vi "一体站流程自动启动.vi"(11 "参数":T1) -> ()   [LabVIEW 2016, in "PLC.lvlib"]
uses:
  PLC.lvlib
panel:
  out "s? t:f":enum16{"初始化", "采配水启动", "仪器操作", "反冲洗", "结束"}(ring)
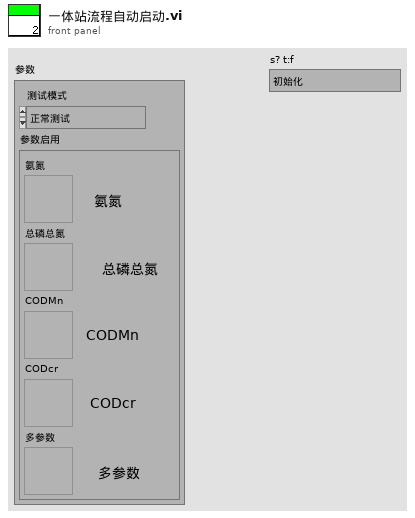
[diagram p1: front panel]
types:
  T1 = cluster{"测试模式":enum16{"正常测试", "集成干预"}, "参数启用":cluster{"氨氮":bool, "总磷总氮":bool, "CODMn":bool, "CODcr":bool, "多参数":bool}}
  T2 = cluster{"命令":string, cluster{"starting address":u16, "holding register value":u16}}
  T3 = enum16{"启动测量", "标样核查", "零点核查", "跨度核查", "空白测试", "平行样测试", "加标回收", "空白校准", "标样校准", "初始化（清洗）", "停止测试", "仪器重启", "校时", "模式设置", "测量间隔设置"}
  T4 = cluster{"时间标识":timestamp, "设备":string, "日志信息":string, "流程参数":string}
  T5 = cluster{"测量模式":enum16{"水样测量", "标样核查", "零点核查", "跨度核查", "空白测试", "加标回收", "平行样", "校零", "校标"}}
  T6 = cluster{"时间标识":timestamp, "设备":string, "日志信息":string}
  T7 = enum16{"空闲", "水样测试", "标样核查", "零点核查", "跨度核查", "空白测试", "平行样测试", "加标回收", "空白校准", "标样校准", "初始化（清洗）"}
  T8 = cluster{"R0":i16, "R1":i16, "R2":i16, "R3":i16, "R4":i16, "R5":i16, "R6":i16, "R7":i16, "R8":i16, "R9":i16, "R10":i16, "R11":i16, "R12":i16, "R13":i16, "R14":i16, "R15":i16, "R16":i16, "R17":i16, "R18":i16, "R19":i16, "R20":i16, "R21":i16, "R22":i16, "R23":i16, "R24":i16, "R25":i16, "R26":i16, "R27":i16, "R28":i16, "R29":i16, "R30":i16, "R31":i16, "R32":i16, "R33":i16, "R34":i16, "R35":i16, "R36":i16, "R37":i16, "R38":i16, "R39":i16, "R40":i16, "R41":i16, "R42":i16, "R43":i16, "R44":i16, "R45":i16, "R46":i16, "R47":i16, "R48":i16, "R49":i16, "R50":i16, "R51":i16, "R52":i16, "R53":i16, "R54":i16, "R55":i16, "R56":i16}
  T9 = cluster{"R100":i16, "R101":i16, "R102":i16, "R103":i16, "R104":i16, "R105":i16, "R106":i16, "R107":i16, "R108":i16, "R109":i16, "R110":i16, "R111":i16, "R112":i16, "R113":i16, "R114":i16, "R115":i16, "R116":i16, "R117":i16, "R118":i16, "R119":i16, "R120":i16, "R121":i16, "R122":i16, "R123":i16}
  T10 = enum32{"Bad", "Idle", "Run top level", "Running"}
  T11 = cluster{"氨氮":bool, "总磷总氮":bool, "CODMn":bool, "CODcr":bool, "多参数":bool}
  T12 = cluster{"时间标识":timestamp, "参数":string, "数据类型":string, "集成干预测试浓度值":dbl, "集成干预前测试时间":timestamp, "集成干预前测试浓度值":dbl}
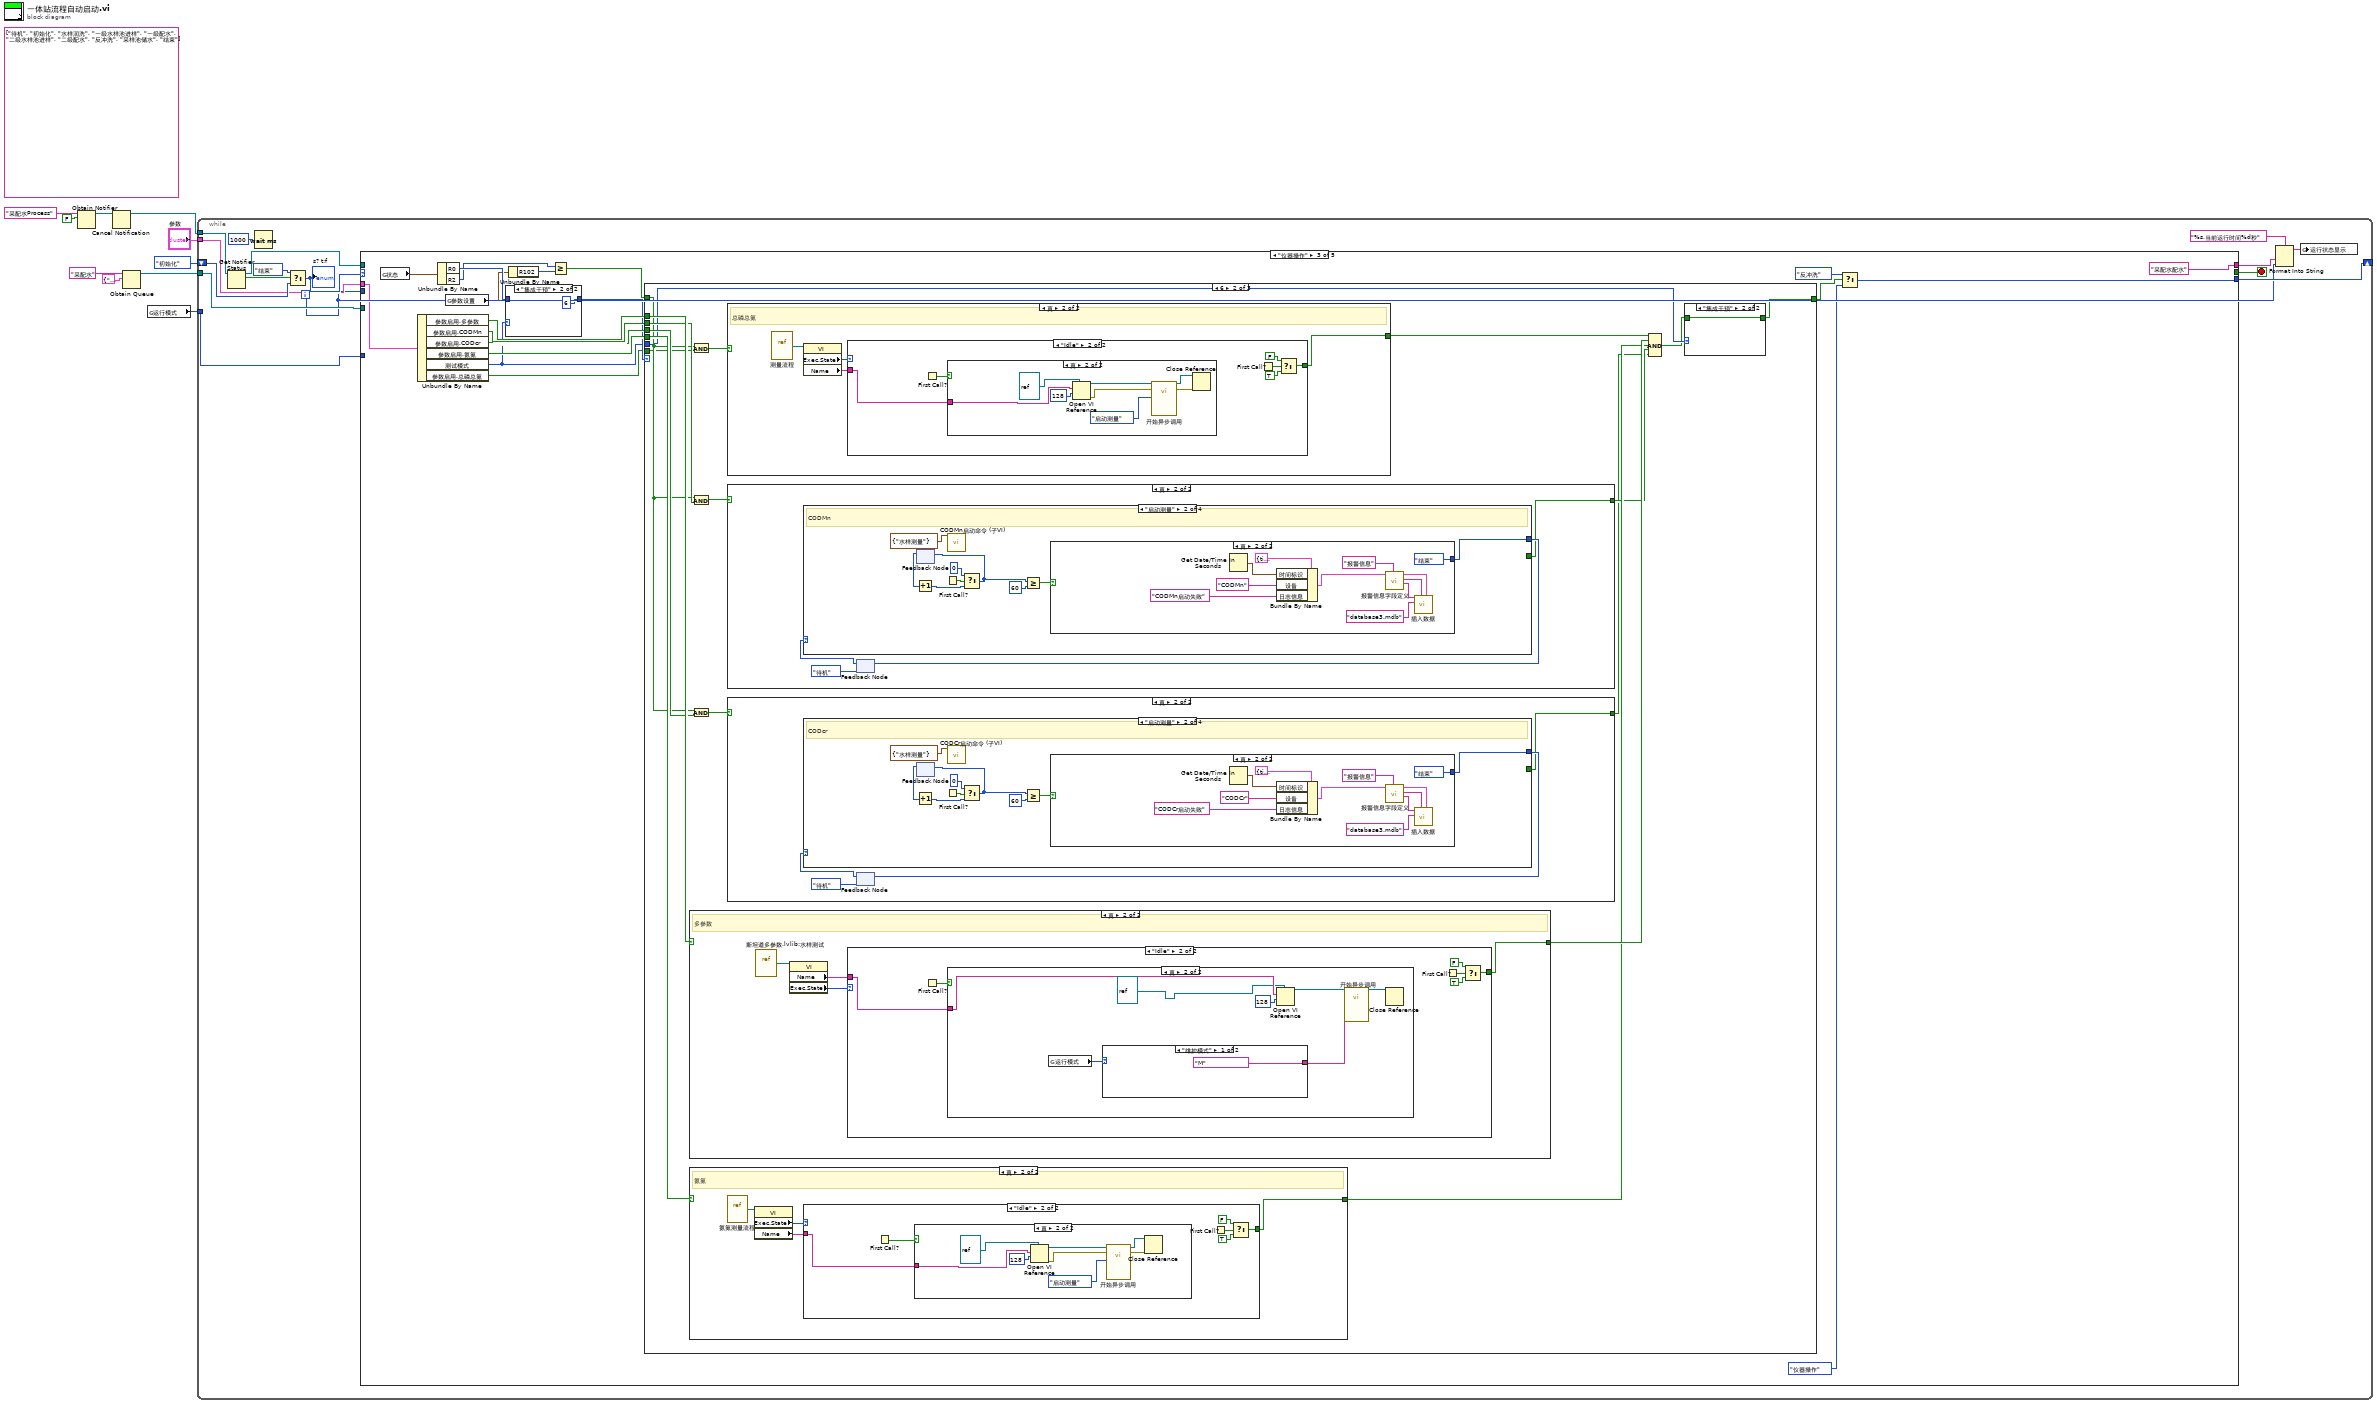
[diagram p0: block diagram]
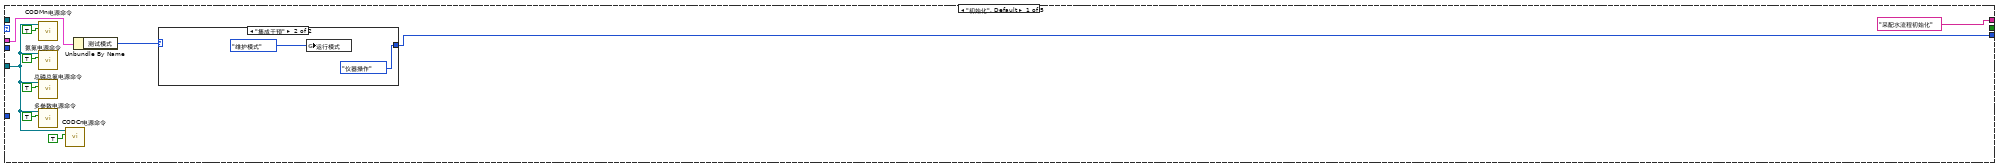
[diagram p2: hidden frame]
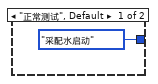
[diagram p3: hidden frame]
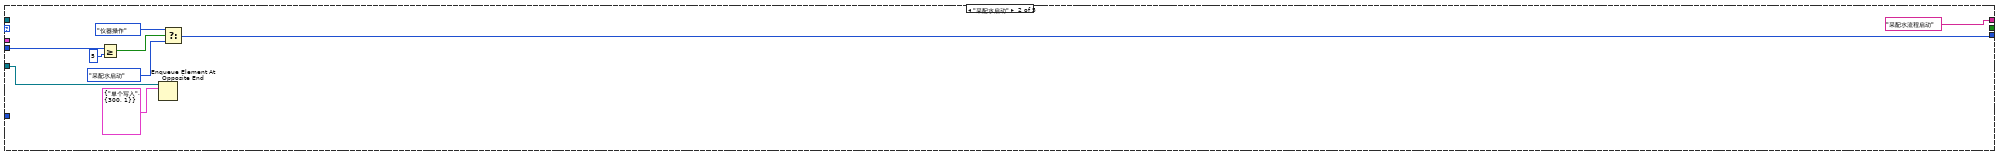
[diagram p4: hidden frame]
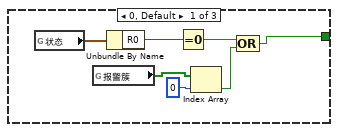
[diagram p6: hidden frame]
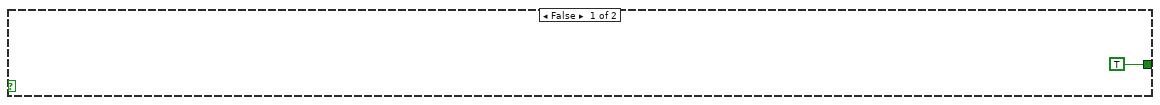
[diagram p7: hidden frame]
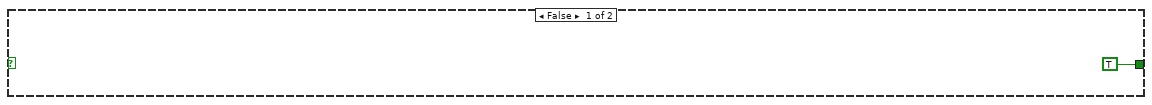
[diagram p11: hidden frame]
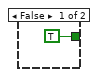
[diagram p14: hidden frame]
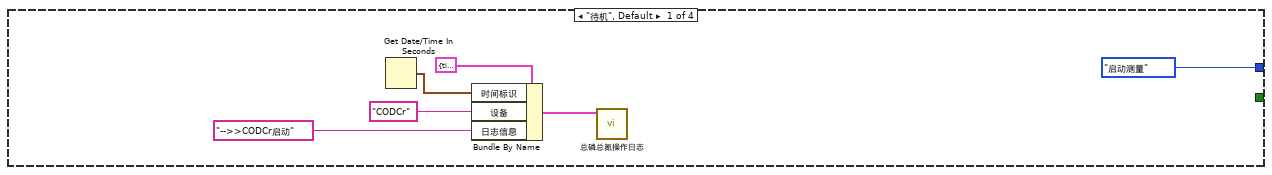
[diagram p15: hidden frame]
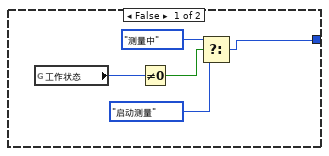
[diagram p16: hidden frame]
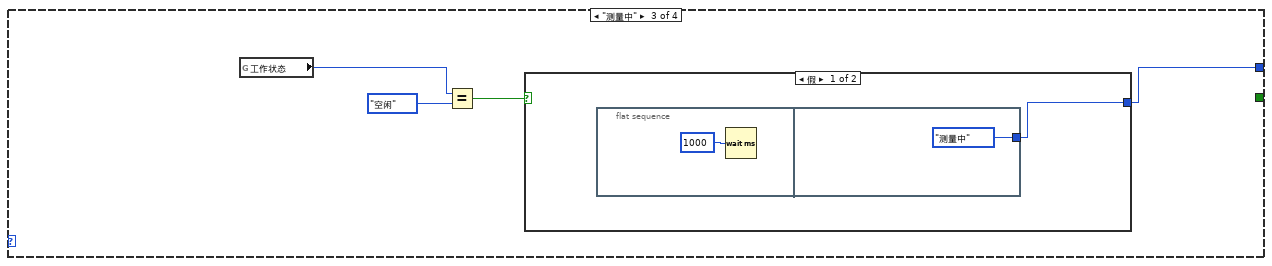
[diagram p17: hidden frame]
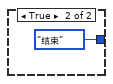
[diagram p18: hidden frame]
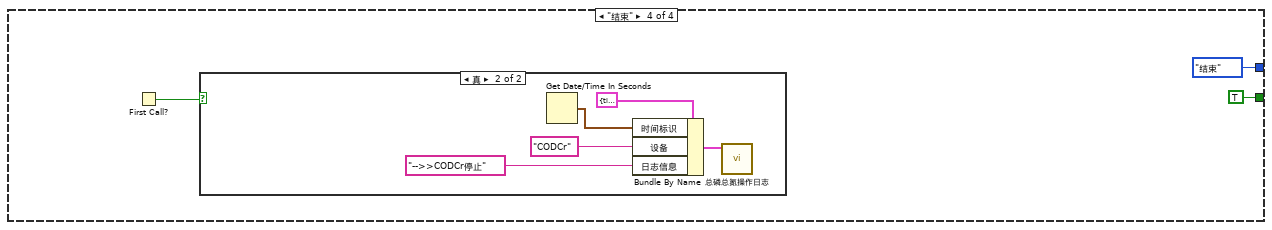
[diagram p19: hidden frame]
diagram:
  (unwired) string[][] [["待机"], ["初始化"], ["水样润洗"], ["一级水样池进样"], ["一级配水"], ["二级水样池进样"], ["二级配水"], ["反冲洗"], ["采样池储水"], ["结束"]] ("项名")
  n1 = Obtain Notifier(name (unnamed)="采配水Process" ("名称（未命名）"), notification data type=FALSE) -> (notifier out=w4:refnum<notifier>)  [unwired: 2 in, 2 out]
  n2 = Cancel Notification(0:w4) -> (8:w3:refnum<notifier>)  [unwired: 1 in, 2 out]
  n3 = Obtain Queue(name (unnamed)="采配水" ("名称（未命名）"), element data type=cluster{"命令":string, "数据":variant} {"命令"="", "数据"=variant}) -> (queue out=w7:refnum<queue>)  [unwired: 3 in, 2 out]
  n4 = global read "系统设置全局变量.vi" "运行模式"() -> (w1:enum16{"维护模式", "常规模式", "应急模式", "质控模式"})
  n5 = while {
    shift-right: [w23] -> _
    shift-left: enum16{"初始化", "采配水启动", "仪器操作", "反冲洗", "结束"}."初始化" ("枚举") -> [w19]
    tunnel: w7 -> [w26]
    tunnel: w3 -> [w22]
    tunnel: "参数" -> [w13]
    tunnel: w1 -> [w12]
    i -> [w11]
    stop <- w25 stop-if-true
    n6 = Get Notifier Status(notifier=w22) -> (notifier out=w14:refnum<notifier>, current notification=w21:bool)  [unwired: 1 in, 3 out]
    n7 = Wait (ms)(milliseconds to wait=u32 1000 ("等待时间（毫秒）")) -> ()  [unwired: 1 out]
    n8 = Select(t=enum16{"初始化", "采配水启动", "仪器操作", "反冲洗", "结束"}."结束" ("枚举"), s=w21, f=w19) -> (s? t:f=w18:enum16{"初始化", "采配水启动", "仪器操作", "反冲洗", "结束"})
    "s? t:f" <- w18
    n9 = case shown="\"仪器操作\"" w18 {
      tunnel: w26 -> [w31 w48 _ _ w434]
      tunnel: [_ _ _ _ TRUE] -> w25
      tunnel: [w30 w40 w62 w261 enum16{"初始化", "采配水启动", "仪器操作", "反冲洗", "结束"}."结束" ("枚举")] -> w23
      tunnel: ["采配水流程初始化" "采配水流程启动" "采配水配水" "等待测试完成" "采配水结束"] -> w15
      tunnel: w14 -> [_ _ _ _ w435]
      tunnel: w13 -> [w28 _ w65 w260 w431]
      tunnel: w12 -> [_ _ _ w257 w430]
      tunnel: w11 -> [_ w46 _ _ _]
      frame "初始化", Default {
        n10 = call "CODMn电源命令.vi"("通电/断电"=TRUE, "队列"=w31) -> ()  [unwired: 9 in, 1 out]
        n11 = call "氨氮电源命令.vi"("通电/断电"=TRUE, "队列"=w31) -> ()  [unwired: 9 in, 1 out]
        n12 = call "总磷总氮电源命令.vi"("通电/断电"=TRUE, "队列"=w31) -> ()  [unwired: 9 in, 1 out]
        n13 = call "多参数电源命令.vi"("通电/断电"=TRUE, "队列"=w31) -> ()  [unwired: 9 in, 1 out]
        n14 = call "CODCr电源命令.vi"("通电/断电"=TRUE, "队列"=w31) -> ()  [unwired: 9 in, 1 out]
        n15 = Unbundle By Name(w28) -> ("测试模式"=w27:enum16{"正常测试", "集成干预"})
        n16 = case shown="\"集成干预\"" w27 {
          tunnel: [enum16{"初始化", "采配水启动", "仪器操作", "反冲洗", "结束"}."采配水启动" ("枚举") enum16{"初始化", "采配水启动", "仪器操作", "反冲洗", "结束"}."仪器操作" ("枚举")] -> w30
          frame "正常测试", Default {
          }
          frame "集成干预" {
            n17 = global write "系统设置全局变量.vi" "运行模式"(enum16{"维护模式", "常规模式", "应急模式", "质控模式"}."维护模式" ("运行模式")) -> ()
          }
        }
      }
      frame "采配水启动" {
        n18 = Greater Or Equal?(x=w46, y=5) -> (x >= y?=w43:bool)
        n19 = Enqueue Element At Opposite End(queue=w48, element=T2 {"命令"="单个写入", {"starting address"=300, "holding register value"=1}} ("元素")) -> ()  [unwired: 2 in, 3 out]
        n20 = Select(t=enum16{"初始化", "采配水启动", "仪器操作", "反冲洗", "结束"}."仪器操作" ("枚举"), s=w43, f=enum16{"初始化", "采配水启动", "仪器操作", "反冲洗", "结束"}."采配水启动" ("枚举")) -> (s? t:f=w40:enum16{"初始化", "采配水启动", "仪器操作", "反冲洗", "结束"})
      }
      frame "仪器操作" {
        n21 = global read "采配水全局变量.vi" "状态"() -> (w67:T8)
        n22 = Unbundle By Name(w65) -> ("参数启用.多参数"=w60:bool, "参数启用.CODMn"=w59:bool, "参数启用.CODcr"=w58:bool, "参数启用.氨氮"=w57:bool, "测试模式"=w50:enum16{"正常测试", "集成干预"}, "参数启用.总磷总氮"=w49:bool)
        n23 = Unbundle By Name(w67) -> ("R0"=w56:i16, "R2"=w51:i16)
        n24 = global read "采配水全局变量.vi" "参数设置"() -> (w53:T9)
        n25 = case shown="\"集成干预\"" w50 {
          tunnel: w56 -> [w68 _]
          tunnel: [w68 i16 6 ("R0")] -> w55
          frame "正常测试", Default {
          }
          frame "集成干预" {
          }
        }
        n26 = Unbundle By Name(w53) -> ("R102"=w54:i16)
        n27 = Greater Or Equal?(x=w51, y=w54) -> (x >= y?=w52:bool)
        n28 = case shown="6" w55 {
          tunnel: [w71 w81 TRUE] -> w64
          tunnel: w60 -> [_ w93 _]
          tunnel: w59 -> [_ w92 _]
          tunnel: w58 -> [_ w89 _]
          tunnel: w57 -> [_ w88 _]
          tunnel: w52 -> [_ w80 _]
          tunnel: w50 -> [_ w83 _]
          tunnel: w49 -> [_ w79 _]
          frame 0, Default {
            n29 = global read "采配水全局变量.vi" "状态"() -> (w74:T8)
            n30 = global read "采配水全局变量.vi" "报警簇"() -> (w75:bool[])
            n31 = Unbundle By Name(w74) -> ("R0"=w73:i16)
            n32 = Equal To 0?(x=w73) -> (x = 0?=w76:bool)
            n33 = Index Array(array=w75, index=0 ("索引")) -> (element=w70:bool)
            n34 = Compound Arithmetic op=OR ("复合运算")(w76, w70) -> (w71:bool)
          }
          frame 6 {
            n35 = case shown="真" w93 {
              tunnel: [TRUE ("t") w237] -> w87
              frame False {
              }
              frame True {
                # "多参数"
                n36 = vi-ref "斯坦道多参数.lvlib:水样测试.vi"() -> (w239:refnum<vi>)
                n37 = property class="VI"(reference=w239) -> ("Name"=w238:string, "Exec.State"=w240:T10)  [unwired: 1 in, 2 out]
                n38 = case shown="\"Idle\"" w240 {
                  tunnel: w238 -> [_ w246]
                  tunnel: [_ w241] -> w237
                  frame "Bad", Default {
                  }
                  frame "Idle" {
                    n39 = First Call?() -> (First Call?: T/F=w245:bool)
                    n40 = case shown="真" w245 {
                      tunnel: w246 -> [_ w252]
                      frame False {
                      }
                      frame True {
                        n41 = global read "系统设置全局变量.vi" "运行模式"() -> (w249:enum16{"维护模式", "常规模式", "应急模式", "质控模式"})
                        n42 = case shown="\"维护模式\"" w249 {
                          tunnel: ["M" ("数据标记表") "N" ("数据标记表")] -> w248
                          frame "维护模式" {
                          }
                          frame "常规模式", Default {
                          }
                        }
                        n43 = Open VI Reference(type specifier VI Refnum (for type only)=refnum<vi> refnum, vi path=w252, options=128 ("选项")) -> (vi reference=w251:refnum<vi>)  [unwired: 3 in, 1 out]
                        n44 = call-by-ref "开始异步调用"(reference=w251, "数据标记表"=w248) -> (reference out=w250:refnum<vi>)  [unwired: 12 in, 1 out]
                        n45 = Close Reference(reference=w250) -> ()  [unwired: 1 in, 1 out]
                      }
                    }
                    n46 = First Call?() -> (First Call?: T/F=w244:bool)
                    n47 = Select(t=FALSE, s=w244, f=TRUE) -> (s? t:f=w241:bool)
                  }
                }
              }
            }
            n48 = case "条件结构" shown="真" w88 {
              tunnel: [TRUE ("t") w115] -> w86
              frame False {
              }
              frame True {
                # "氨氮"
                n49 = vi-ref "氨氮测量流程.vi"() -> (w118:refnum<vi>)
                n50 = property class="VI"(reference=w118) -> ("Exec.State"=w117:T10, "Name"=w116:string)  [unwired: 1 in, 2 out]
                n51 = case shown="\"Idle\"" w117 {
                  tunnel: w116 -> [_ w124]
                  tunnel: [_ w119] -> w115
                  frame "Bad", Default {
                  }
                  frame "Idle" {
                    n52 = First Call?() -> (First Call?: T/F=w123:bool)
                    n53 = case shown="真" w123 {
                      tunnel: w124 -> [_ w129]
                      frame False {
                      }
                      frame True {
                        n54 = Open VI Reference(type specifier VI Refnum (for type only)=refnum<vi> refnum, vi path=w129, options=128 ("选项")) -> (vi reference=w127:refnum<vi>, error out=w130:errorcluster)  [unwired: 3 in]
                        n55 = call-by-ref "开始异步调用"(reference=w127, error in=w130, "控制命令"=T3."启动测量") -> (reference out=w131:refnum<vi>, error out=w132:errorcluster)  [unwired: 11 in]
                        n56 = Close Reference(reference=w131, error in (no error)=w132) -> ()  [unwired: 1 out]
                      }
                    }
                    n57 = First Call?() -> (First Call?: T/F=w122:bool)
                    n58 = Select(t=FALSE, s=w122, f=TRUE) -> (s? t:f=w119:bool)
                  }
                }
              }
            }
            n59 = And(x=w80, y=w79) -> (x .and. y?=w78:bool)
            n60 = And(x=w80, y=w92) -> (x .and. y?=w91:bool)
            n61 = And(x=w80, y=w89) -> (x .and. y?=w90:bool)
            n62 = case "条件结构" shown="真" w78 {
              tunnel: [TRUE ("t") w95] -> w77
              frame False {
              }
              frame True {
                # "总磷总氮"
                n63 = vi-ref "测量流程.vi"() -> (w98:refnum<vi>)
                n64 = property class="VI"(reference=w98) -> ("Exec.State"=w97:T10, "Name"=w96:string)  [unwired: 1 in, 2 out]
                n65 = case shown="\"Idle\"" w97 {
                  tunnel: w96 -> [_ w104]
                  tunnel: [_ w99] -> w95
                  frame "Bad", Default {
                  }
                  frame "Idle" {
                    n66 = First Call?() -> (First Call?: T/F=w103:bool)
                    n67 = case shown="真" w103 {
                      tunnel: w104 -> [_ w109]
                      frame False {
                      }
                      frame True {
                        n68 = Open VI Reference(type specifier VI Refnum (for type only)=refnum<vi> refnum, vi path=w109, options=128 ("选项")) -> (vi reference=w107:refnum<vi>, error out=w110:errorcluster)  [unwired: 3 in]
                        n69 = call-by-ref "开始异步调用"(reference=w107, error in=w110, "控制命令"=T3."启动测量") -> (reference out=w111:refnum<vi>, error out=w112:errorcluster)  [unwired: 11 in]
                        n70 = Close Reference(reference=w111, error in (no error)=w112) -> ()  [unwired: 1 out]
                      }
                    }
                    n71 = First Call?() -> (First Call?: T/F=w102:bool)
                    n72 = Select(t=FALSE, s=w102, f=TRUE) -> (s? t:f=w99:bool)
                  }
                }
              }
            }
            n73 = case shown="真" w91 {
              tunnel: [TRUE w186] -> w85
              frame False {
              }
              frame True {
                n74 = feedback #1(enum16{"待机", "启动测量", "测量中", "结束"}."待机") -> (w188:enum16{"待机", "启动测量", "测量中", "结束"})
                n75 = case shown="\"启动测量\"" w188 {
                  tunnel: [enum16{"待机", "启动测量", "测量中", "结束"}."启动测量" w204 w223 enum16{"待机", "启动测量", "测量中", "结束"}."结束"] -> w187
                  tunnel: [_ _ _ TRUE] -> w186
                  frame "待机", Default {
                    n76 = Get Date/Time In Seconds() -> (seconds since 1Jan1904=w194:timestamp)
                    n77 = Bundle By Name(cluster=T4 {"时间标识"=timestamp(0 s since 1904-01-01), "设备"="", "日志信息"="", "流程参数"=""} ("data in"), "时间标识"=w194, "设备"="CODMn", "日志信息"="-->>CODMn启动") -> (w190:T4)
                    n78 = call "总磷总氮操作日志.vi"("data in"=w190) -> ()  [unwired: 11 in]
                  }
                  frame "启动测量" {
                    # "CODMn"
                    n79 = feedback #2() -> (w200:i32)  [unwired: 1 in]
                    n80 = Increment(x=w200) -> (x+1=w201:i32)
                    n81 = First Call?() -> (First Call?: T/F=w199:bool)
                    n82 = call "CODMn启动命令 (子VI).vi"("启动测量模式"=T5 {"测量模式"=enum."水样测量"}) -> ()  [unwired: 11 in]
                    n83 = Select(t=0, s=w199, f=w201) -> (s? t:f=w202:i32)
                    n84 = feedback-in #2(w202) -> ()
                    n85 = Greater Or Equal?(x=w202, y=60) -> (x >= y?=w197:bool)
                    n86 = case shown="真" w197 {
                      tunnel: [w206 enum16{"待机", "启动测量", "测量中", "结束"}."结束"] -> w204
                      frame False {
                        n87 = global read "运行时序全局变量.vi" "多列列表框"() -> (w205:i32)
                        n88 = Not Equal To 0?(x=w205) -> (x != 0?=w207:bool)
                        n89 = Select(t=enum16{"待机", "启动测量", "测量中", "结束"}."测量中", s=w207, f=enum16{"待机", "启动测量", "测量中", "结束"}."启动测量") -> (s? t:f=w206:enum16{"待机", "启动测量", "测量中", "结束"})
                      }
                      frame True {
                        n90 = Get Date/Time In Seconds() -> (seconds since 1Jan1904=w216:timestamp)
                        n91 = Bundle By Name(cluster=T6 {"时间标识"=timestamp(0 s since 1904-01-01), "设备"="", "日志信息"=""} ("data in"), "时间标识"=w216, "设备"="CODMn", "日志信息"="CODMn启动失败") -> (w210:T6)
                        n92 = call "报警信息字段定义.vi"("table输入"="报警信息", "data in"=w210) -> ("table输出"=w213:string, "columns"=w214:string[], "data out"=w215:T6)  [unwired: 7 in]
                        n93 = call "插入数据.vi"("data"=w215, "columns"=w214, "database"="database3.mdb", "table"=w213) -> ()  [unwired: 7 in, 1 out]
                      }
                    }
                  }
                  frame "测量中" {
                    n94 = global read "运行时序全局变量.vi" "多列列表框"() -> (w222:i32)
                    n95 = Equal To 0?(x=w222) -> (x = 0?=w221:bool)
                    n96 = case shown="假" w221 {
                      tunnel: [w224 enum16{"待机", "启动测量", "测量中", "结束"}."结束"] -> w223
                      frame False {
                        n97 = flat-sequence {
                          tunnel: [enum16{"待机", "启动测量", "测量中", "结束"}."测量中"] -> w224
                          frame #0 {
                            n98 = Wait (ms)(milliseconds to wait=u32 1000 ("等待时间（毫秒）")) -> ()  [unwired: 1 out]
                          }
                          frame #1 {
                          }
                        }
                      }
                      frame True {
                      }
                    }
                  }
                  frame "结束" {
                    n99 = First Call?() -> (First Call?: T/F=w228:bool)
                    n100 = case shown="真" w228 {
                      frame False {
                      }
                      frame True {
                        n101 = Get Date/Time In Seconds() -> (seconds since 1Jan1904=w235:timestamp)
                        n102 = Bundle By Name(cluster=T4 {"时间标识"=timestamp(0 s since 1904-01-01), "设备"="", "日志信息"="", "流程参数"=""} ("data in"), "时间标识"=w235, "设备"="CODMn", "日志信息"="-->>CODMn停止") -> (w231:T4)
                        n103 = call "总磷总氮操作日志.vi"("data in"=w231) -> ()  [unwired: 11 in]
                      }
                    }
                  }
                }
                n104 = feedback-in #1(w187) -> ()
              }
            }
            n105 = case shown="真" w90 {
              tunnel: [TRUE w134] -> w84
              frame False {
              }
              frame True {
                n106 = feedback #3(enum16{"待机", "启动测量", "测量中", "结束"}."待机") -> (w136:enum16{"待机", "启动测量", "测量中", "结束"})
                n107 = case shown="\"启动测量\"" w136 {
                  tunnel: [enum16{"待机", "启动测量", "测量中", "结束"}."启动测量" w152 w172 enum16{"待机", "启动测量", "测量中", "结束"}."结束"] -> w135
                  tunnel: [_ _ _ TRUE] -> w134
                  frame "待机", Default {
                    n108 = Get Date/Time In Seconds() -> (seconds since 1Jan1904=w142:timestamp)
                    n109 = Bundle By Name(cluster=T4 {"时间标识"=timestamp(0 s since 1904-01-01), "设备"="", "日志信息"="", "流程参数"=""} ("data in"), "时间标识"=w142, "设备"="CODCr", "日志信息"="-->>CODCr启动") -> (w138:T4)
                    n110 = call "总磷总氮操作日志.vi"("data in"=w138) -> ()  [unwired: 11 in]
                  }
                  frame "启动测量" {
                    # "CODcr"
                    n111 = feedback #4() -> (w148:i32)  [unwired: 1 in]
                    n112 = Increment(x=w148) -> (x+1=w149:i32)
                    n113 = First Call?() -> (First Call?: T/F=w147:bool)
                    n114 = call "CODCr启动命令 (子VI).vi"("启动测量模式"=T5 {"测量模式"=enum."水样测量"}) -> ()  [unwired: 11 in]
                    n115 = Select(t=0, s=w147, f=w149) -> (s? t:f=w150:i32)
                    n116 = feedback-in #4(w150) -> ()
                    n117 = Greater Or Equal?(x=w150, y=60) -> (x >= y?=w145:bool)
                    n118 = case shown="真" w145 {
                      tunnel: [w153 enum16{"待机", "启动测量", "测量中", "结束"}."结束"] -> w152
                      frame False {
                        n119 = global read "CODcr全局变量.vi" "工作状态"() -> (w154:T7)
                        n120 = Not Equal To 0?(x=w154) -> (x != 0?=w155:bool)
                        n121 = Select(t=enum16{"待机", "启动测量", "测量中", "结束"}."测量中", s=w155, f=enum16{"待机", "启动测量", "测量中", "结束"}."启动测量") -> (s? t:f=w153:enum16{"待机", "启动测量", "测量中", "结束"})
                      }
                      frame True {
                        n122 = Get Date/Time In Seconds() -> (seconds since 1Jan1904=w164:timestamp)
                        n123 = Bundle By Name(cluster=T6 {"时间标识"=timestamp(0 s since 1904-01-01), "设备"="", "日志信息"=""} ("data in"), "时间标识"=w164, "设备"="CODCr", "日志信息"="CODCr启动失败") -> (w158:T6)
                        n124 = call "报警信息字段定义.vi"("table输入"="报警信息", "data in"=w158) -> ("table输出"=w161:string, "columns"=w162:string[], "data out"=w163:T6)  [unwired: 7 in]
                        n125 = call "插入数据.vi"("data"=w163, "columns"=w162, "database"="database3.mdb", "table"=w161) -> ()  [unwired: 7 in, 1 out]
                      }
                    }
                  }
                  frame "测量中" {
                    n126 = global read "CODcr全局变量.vi" "工作状态"() -> (w171:T7)
                    n127 = Equal?(x=w171, y=T7."空闲" ("工作状态")) -> (x = y?=w170:bool)
                    n128 = case shown="假" w170 {
                      tunnel: [w173 enum16{"待机", "启动测量", "测量中", "结束"}."结束"] -> w172
                      frame False {
                        n129 = flat-sequence {
                          tunnel: [enum16{"待机", "启动测量", "测量中", "结束"}."测量中"] -> w173
                          frame #0 {
                            n130 = Wait (ms)(milliseconds to wait=u32 1000 ("等待时间（毫秒）")) -> ()  [unwired: 1 out]
                          }
                          frame #1 {
                          }
                        }
                      }
                      frame True {
                      }
                    }
                  }
                  frame "结束" {
                    n131 = First Call?() -> (First Call?: T/F=w177:bool)
                    n132 = case shown="真" w177 {
                      frame False {
                      }
                      frame True {
                        n133 = Get Date/Time In Seconds() -> (seconds since 1Jan1904=w184:timestamp)
                        n134 = Bundle By Name(cluster=T4 {"时间标识"=timestamp(0 s since 1904-01-01), "设备"="", "日志信息"="", "流程参数"=""} ("data in"), "时间标识"=w184, "设备"="CODCr", "日志信息"="-->>CODCr停止") -> (w180:T4)
                        n135 = call "总磷总氮操作日志.vi"("data in"=w180) -> ()  [unwired: 11 in]
                      }
                    }
                  }
                }
                n136 = feedback-in #3(w135) -> ()
              }
            }
            n137 = Compound Arithmetic op=AND ("复合运算")(w77, w87, w86, w85, w84) -> (w82:bool)
            n138 = case shown="\"集成干预\"" w83 {
              tunnel: w82 -> [_ w113]
              tunnel: [_ w113] -> w81
              frame "正常测试", Default {
              }
              frame "集成干预" {
              }
            }
          }
          frame 7..9 {
          }
        }
        n139 = Select(t=enum16{"初始化", "采配水启动", "仪器操作", "反冲洗", "结束"}."反冲洗" ("枚举"), s=w64, f=enum16{"初始化", "采配水启动", "仪器操作", "反冲洗", "结束"}."仪器操作" ("枚举")) -> (s? t:f=w62:enum16{"初始化", "采配水启动", "仪器操作", "反冲洗", "结束"})
      }
      frame "反冲洗" {
        n140 = First Call?() -> (First Call?: T/F=w258:bool)
        n141 = case shown="真" w258 {
          tunnel: w260 -> [_ w270]
          tunnel: w257 -> [_ w267]
          frame False {
          }
          frame True {
            n142 = Unbundle By Name(w270) -> ("测试模式"=w269:enum16{"正常测试", "集成干预"}, "参数启用"=w268:T11)
            n143 = case shown="\"集成干预\"" w269 {
              tunnel: w268 -> [w273 w358]
              tunnel: w267 -> [_ w353]
              frame "正常测试", Default {
                n144 = global read "系统设置全局变量.vi" "运行模式"() -> (w271:enum16{"维护模式", "常规模式", "应急模式", "质控模式"})
                n145 = global read "采配水全局变量.vi" "报警簇"() -> (w278:bool[])
                n146 = case shown="\"维护模式\"" w271 {
                  tunnel: ["M" ("table") "N" ("table")] -> w272
                  frame "维护模式" {
                  }
                  frame "常规模式", Default {
                  }
                }
                n147 = Index Array(array=w278, index #1=0 ("索引"), index #2=11 ("索引")) -> (element #1=w275:bool, element #2=w274:bool)
                n148 = case shown="假" w275 {
                  tunnel: w274 -> [w284 _]
                  tunnel: w273 -> [w283 w297]
                  tunnel: w272 -> [w281 w291]
                  frame False {
                    n149 = Unbundle By Name(w283) -> ("氨氮"=w282:bool)
                    n150 = case shown="真" w284 {
                      tunnel: w282 -> [_ w286]
                      tunnel: w281 -> [_ w285]
                      frame False {
                      }
                      frame True {
                        n151 = case shown="真" w286 {
                          tunnel: w285 -> [_ w287]
                          tunnel: [_ w288] -> _
                          frame False {
                          }
                          frame True {
                            n152 = call "取水点无水样数据存储.vi"("数据标识"="lw", "数据类型"=w287, "table"="氨氮") -> ("error out"=w288:errorcluster)  [unwired: 8 in]
                          }
                        }
                      }
                    }
                  }
                  frame True {
                    n153 = Unbundle By Name(w297) -> ("氨氮"=w296:bool, "CODMn"=w295:bool, "CODcr"=w294:bool, "多参数"=w293:bool, "总磷总氮"=w292:bool)
                    n154 = case shown="真" w296 {
                      tunnel: w291 -> [_ w349]
                      tunnel: [_ w350] -> _
                      frame False {
                      }
                      frame True {
                        n155 = call "取水点无水样数据存储.vi"("数据标识"="Z", "数据类型"=w349, "table"="氨氮") -> ("error out"=w350:errorcluster)  [unwired: 8 in]
                      }
                    }
                    n156 = case shown="真" w295 {
                      tunnel: w291 -> [_ w346]
                      tunnel: [_ w345] -> _
                      frame False {
                      }
                      frame True {
                        n157 = call "取水点无水样数据存储.vi"("数据标识"="Z", "数据类型"=w346, "table"="CODMn") -> ("error out"=w345:errorcluster)  [unwired: 8 in]
                      }
                    }
                    n158 = case shown="真" w294 {
                      tunnel: w291 -> [_ w342]
                      tunnel: [_ w341] -> _
                      frame False {
                      }
                      frame True {
                        n159 = call "取水点无水样数据存储.vi"("数据标识"="Z", "数据类型"=w342, "table"="CODCr") -> ("error out"=w341:errorcluster)  [unwired: 8 in]
                      }
                    }
                    n160 = case shown="真" w292 {
                      tunnel: w291 -> [_ w299]
                      tunnel: [_ w298] -> _
                      frame False {
                      }
                      frame True {
                        n161 = call "取水点无水样数据存储.vi"("数据标识"="Z", "数据类型"=w299, "table"="总氮") -> ("error out"=w300:errorcluster)  [unwired: 8 in]
                        n162 = call "取水点无水样数据存储.vi"("error in (no error)"=w300, "数据标识"="Z", "数据类型"=w299, "table"="总磷") -> ("error out"=w298:errorcluster)  [unwired: 7 in]
                      }
                    }
                    n163 = case shown="真" w293 {
                      tunnel: w291 -> [_ w312]
                      frame False {
                      }
                      frame True {
                        n164 = global read "断电保存变量.vi" "Cond"() -> (w307:bool)
                        n165 = global read "断电保存变量.vi" "Turb"() -> (w308:bool)
                        n166 = global read "断电保存变量.vi" "DO"() -> (w309:bool)
                        n167 = global read "断电保存变量.vi" "pH"() -> (w310:bool)
                        n168 = global read "断电保存变量.vi" "藻密度"() -> (w306:bool)
                        n169 = global read "断电保存变量.vi" "Temp"() -> (w311:bool)
                        n170 = case shown="真" w310 {
                          tunnel: w312 -> [_ w334]
                          tunnel: [_ w333] -> _
                          frame False {
                          }
                          frame True {
                            n171 = call "取水点无水样数据存储.vi"("数据标识"="Z", "数据类型"=w334, "table"="pH") -> ("error out"=w333:errorcluster)  [unwired: 8 in]
                          }
                        }
                        n172 = case shown="真" w309 {
                          tunnel: w312 -> [_ w330]
                          tunnel: [_ w329] -> _
                          frame False {
                          }
                          frame True {
                            n173 = call "取水点无水样数据存储.vi"("数据标识"="Z", "数据类型"=w330, "table"="DO") -> ("error out"=w329:errorcluster)  [unwired: 8 in]
                          }
                        }
                        n174 = case shown="真" w308 {
                          tunnel: w312 -> [_ w322]
                          tunnel: [_ w321] -> _
                          frame False {
                          }
                          frame True {
                            n175 = call "取水点无水样数据存储.vi"("数据标识"="Z", "数据类型"=w322, "table"="浊度") -> ("error out"=w321:errorcluster)  [unwired: 8 in]
                          }
                        }
                        n176 = case shown="真" w307 {
                          tunnel: w312 -> [_ w326]
                          tunnel: [_ w325] -> _
                          frame False {
                          }
                          frame True {
                            n177 = call "取水点无水样数据存储.vi"("数据标识"="Z", "数据类型"=w326, "table"="比电导率") -> ("error out"=w325:errorcluster)  [unwired: 8 in]
                          }
                        }
                        n178 = global read "断电保存变量.vi" "叶绿素a启用"() -> (w305:bool)
                        n179 = case shown="真" w311 {
                          tunnel: w312 -> [_ w338]
                          tunnel: [_ w337] -> _
                          frame False {
                          }
                          frame True {
                            n180 = call "取水点无水样数据存储.vi"("数据标识"="Z", "数据类型"=w338, "table"="水温") -> ("error out"=w337:errorcluster)  [unwired: 8 in]
                          }
                        }
                        n181 = case shown="真" w306 {
                          tunnel: w312 -> [_ w314]
                          tunnel: [_ w313] -> _
                          frame False {
                          }
                          frame True {
                            n182 = call "取水点无水样数据存储.vi"("数据标识"="Z", "数据类型"=w314, "table"="藻密度") -> ("error out"=w313:errorcluster)  [unwired: 8 in]
                          }
                        }
                        n183 = case shown="真" w305 {
                          tunnel: w312 -> [_ w318]
                          tunnel: [_ w317] -> _
                          frame False {
                          }
                          frame True {
                            n184 = call "取水点无水样数据存储.vi"("数据标识"="Z", "数据类型"=w318, "table"="叶绿素a") -> ("error out"=w317:errorcluster)  [unwired: 8 in]
                          }
                        }
                      }
                    }
                  }
                }
              }
              frame "集成干预" {
                n185 = Unbundle By Name(w358) -> ("氨氮"=w357:bool, "CODMn"=w356:bool, "CODcr"=w355:bool, "多参数"=w354:bool)
                n186 = case shown="真" w357 {
                  tunnel: w353 -> [_ w422]
                  frame False {
                  }
                  frame True {
                    n187 = call "获取最近两组水样测试数据.vi"("运行模式"=w422, "table"="氨氮") -> ("error out"=w427:errorcluster, "存储变量"=w428:T12)  [unwired: 8 in]
                    n188 = call "集成干预测试数据存储.vi"("error in (no error)"=w427, "存储变量"=w428) -> ("error out"=w423:errorcluster)  [unwired: 9 in]
                    n189 = call "获取最近两组水样测试数据.vi"("error in (no error)"=w423, "运行模式"=w422, "table"="总磷") -> ("error out"=w426:errorcluster, "存储变量"=w425:T12)  [unwired: 7 in]
                    n190 = call "集成干预测试数据存储.vi"("error in (no error)"=w426, "存储变量"=w425) -> ()  [unwired: 9 in, 1 out]
                  }
                }
                n191 = case shown="真" w356 {
                  tunnel: w353 -> [_ w418]
                  frame False {
                  }
                  frame True {
                    n192 = call "获取最近两组水样测试数据.vi"("运行模式"=w418, "table"="CODMn") -> ("error out"=w419:errorcluster, "存储变量"=w420:T12)  [unwired: 8 in]
                    n193 = call "集成干预测试数据存储.vi"("error in (no error)"=w419, "存储变量"=w420) -> ()  [unwired: 9 in, 1 out]
                  }
                }
                n194 = case shown="真" w355 {
                  tunnel: w353 -> [_ w414]
                  frame False {
                  }
                  frame True {
                    n195 = call "获取最近两组水样测试数据.vi"("运行模式"=w414, "table"="CODCr") -> ("error out"=w415:errorcluster, "存储变量"=w416:T12)  [unwired: 8 in]
                    n196 = call "集成干预测试数据存储.vi"("error in (no error)"=w415, "存储变量"=w416) -> ()  [unwired: 9 in, 1 out]
                  }
                }
                n197 = case shown="真" w354 {
                  tunnel: w353 -> [_ w359]
                  frame False {
                  }
                  frame True {
                    n198 = global read "断电保存变量.vi" "Temp"() -> (w366:bool)
                    n199 = case shown="真" w366 {
                      tunnel: [_ w410] -> w372
                      tunnel: w359 -> [_ w409]
                      frame False {
                      }
                      frame True {
                        n200 = call "获取最近两组水样测试数据.vi"("运行模式"=w409, "table"="水温") -> ("error out"=w413:errorcluster, "存储变量"=w412:T12)  [unwired: 8 in]
                        n201 = call "集成干预测试数据存储.vi"("error in (no error)"=w413, "存储变量"=w412) -> ("error out"=w410:errorcluster)  [unwired: 9 in]
                      }
                    }
                    n202 = global read "断电保存变量.vi" "pH"() -> (w365:bool)
                    n203 = case shown="真" w365 {
                      tunnel: [_ w405] -> w371
                      tunnel: w372 -> [_ w404]
                      tunnel: w359 -> [_ w403]
                      frame False {
                      }
                      frame True {
                        n204 = call "获取最近两组水样测试数据.vi"("error in (no error)"=w404, "运行模式"=w403, "table"="pH") -> ("error out"=w408:errorcluster, "存储变量"=w407:T12)  [unwired: 7 in]
                        n205 = call "集成干预测试数据存储.vi"("error in (no error)"=w408, "存储变量"=w407) -> ("error out"=w405:errorcluster)  [unwired: 9 in]
                      }
                    }
                    n206 = global read "断电保存变量.vi" "DO"() -> (w364:bool)
                    n207 = case shown="真" w364 {
                      tunnel: [_ w399] -> w370
                      tunnel: w371 -> [_ w398]
                      tunnel: w359 -> [_ w397]
                      frame False {
                      }
                      frame True {
                        n208 = call "获取最近两组水样测试数据.vi"("error in (no error)"=w398, "运行模式"=w397, "table"="DO") -> ("error out"=w402:errorcluster, "存储变量"=w401:T12)  [unwired: 7 in]
                        n209 = call "集成干预测试数据存储.vi"("error in (no error)"=w402, "存储变量"=w401) -> ("error out"=w399:errorcluster)  [unwired: 9 in]
                      }
                    }
                    n210 = global read "断电保存变量.vi" "Cond"() -> (w363:bool)
                    n211 = case shown="真" w363 {
                      tunnel: [_ w393] -> w369
                      tunnel: w370 -> [_ w392]
                      tunnel: w359 -> [_ w391]
                      frame False {
                      }
                      frame True {
                        n212 = call "获取最近两组水样测试数据.vi"("error in (no error)"=w392, "运行模式"=w391, "table"="电导率") -> ("error out"=w396:errorcluster, "存储变量"=w395:T12)  [unwired: 7 in]
                        n213 = call "集成干预测试数据存储.vi"("error in (no error)"=w396, "存储变量"=w395) -> ("error out"=w393:errorcluster)  [unwired: 9 in]
                      }
                    }
                    n214 = global read "断电保存变量.vi" "Turb"() -> (w362:bool)
                    n215 = case shown="真" w362 {
                      tunnel: [_ w387] -> w368
                      tunnel: w369 -> [_ w386]
                      tunnel: w359 -> [_ w385]
                      frame False {
                      }
                      frame True {
                        n216 = call "获取最近两组水样测试数据.vi"("error in (no error)"=w386, "运行模式"=w385, "table"="浊度") -> ("error out"=w390:errorcluster, "存储变量"=w389:T12)  [unwired: 7 in]
                        n217 = call "集成干预测试数据存储.vi"("error in (no error)"=w390, "存储变量"=w389) -> ("error out"=w387:errorcluster)  [unwired: 9 in]
                      }
                    }
                    n218 = global read "断电保存变量.vi" "叶绿素a启用"() -> (w361:bool)
                    n219 = case shown="真" w361 {
                      tunnel: [_ w381] -> w367
                      tunnel: w368 -> [_ w380]
                      tunnel: w359 -> [_ w379]
                      frame False {
                      }
                      frame True {
                        n220 = call "获取最近两组水样测试数据.vi"("error in (no error)"=w380, "运行模式"=w379, "table"="叶绿素a") -> ("error out"=w384:errorcluster, "存储变量"=w383:T12)  [unwired: 7 in]
                        n221 = call "集成干预测试数据存储.vi"("error in (no error)"=w384, "存储变量"=w383) -> ("error out"=w381:errorcluster)  [unwired: 9 in]
                      }
                    }
                    n222 = global read "断电保存变量.vi" "藻密度"() -> (w360:bool)
                    n223 = case shown="真" w360 {
                      tunnel: [_ w375] -> _
                      tunnel: w367 -> [_ w374]
                      tunnel: w359 -> [_ w373]
                      frame False {
                      }
                      frame True {
                        n224 = call "获取最近两组水样测试数据.vi"("error in (no error)"=w374, "运行模式"=w373, "table"="藻密度") -> ("error out"=w378:errorcluster, "存储变量"=w377:T12)  [unwired: 7 in]
                        n225 = call "集成干预测试数据存储.vi"("error in (no error)"=w378, "存储变量"=w377) -> ("error out"=w375:errorcluster)  [unwired: 9 in]
                      }
                    }
                  }
                }
              }
            }
          }
        }
        n226 = global read "采配水全局变量.vi" "状态"() -> (w266:T8)
        n227 = Unbundle By Name(w266) -> ("R0"=w265:i16)
        n228 = Equal To 0?(x=w265) -> (x = 0?=w264:bool)
        n229 = Select(t=enum16{"初始化", "采配水启动", "仪器操作", "反冲洗", "结束"}."结束" ("枚举"), s=w264, f=enum16{"初始化", "采配水启动", "仪器操作", "反冲洗", "结束"}."反冲洗" ("枚举")) -> (s? t:f=w261:enum16{"初始化", "采配水启动", "仪器操作", "反冲洗", "结束"})
      }
      frame "结束" {
        n230 = Release Queue(queue=w434) -> ()  [unwired: 2 in, 3 out]
        n231 = Unbundle By Name(w431) -> ("测试模式"=w432:enum16{"正常测试", "集成干预"})
        n232 = Cancel Notification(0:w435) -> (8:w436:refnum<notifier>)  [unwired: 1 in, 2 out]
        n233 = Release Notifier(notifier=w436) -> ()  [unwired: 2 in, 3 out]
        n234 = case shown="\"集成干预\"" w432 {
          tunnel: w430 -> [_ w439]
          frame "正常测试", Default {
          }
          frame "集成干预" {
            n235 = global write "系统设置全局变量.vi" "运行模式"(w439) -> ()
          }
        }
      }
    }
    n236 = Format Into String(format string="%s,当前运行时间%d秒" ("格式字符串"), w15, w11) -> (resulting string=w16:string)  [unwired: 2 in, 1 out]
    n237 = global write "采配水全局变量.vi" "运行状态显示"(w16) -> ()
  }
